vi "onPrevious.vi"(8 "error in (no error)":errorcluster, 10 "Player In":refnum<class "Player.lvclass">, 11 "PlayingState in":refnum<class "PlayingState.lvclass">) -> (0 "error out":errorcluster, 1 "String":string, 2 "Player Out":refnum<class "Player.lvclass">, 3 "PlayingState out":refnum<class "PlayingState.lvclass">)   [LabVIEW 2017, in "PlayingState.lvclass"]
uses:
  PlayingState.lvclass
  Player Class/Player.lvclass
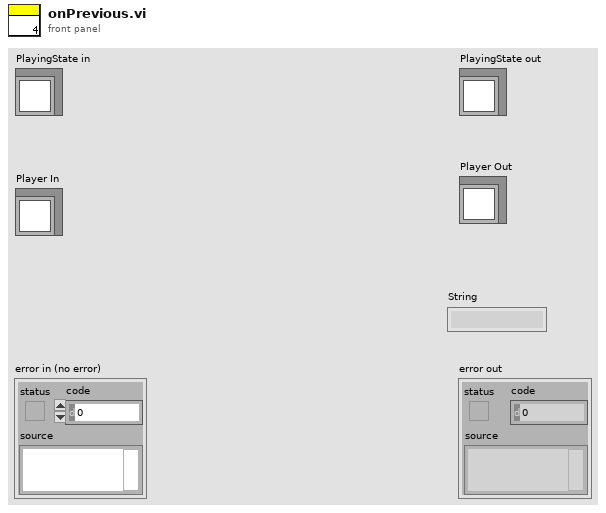
[diagram p1: front panel]
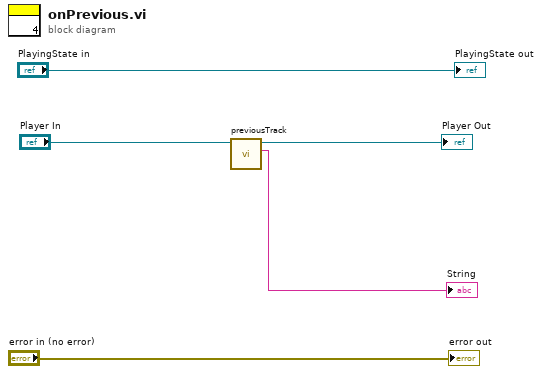
[diagram p0: block diagram]
diagram:
  n1 = call-dynamic "previousTrack.vi"("Player in"="Player In") -> ("Song"=→"String":string, "Player out"=→"Player Out":refnum<class "Player.lvclass">)  [unwired: 8 in, 1 out]
  "error out" <- "error in (no error)"
  "PlayingState out" <- "PlayingState in"
